vi "ConfigureChannelTrigger.vi"(8 "Error In":errorcluster, 10 "Channel Configuration":T1, 11 "Keithley 7001 In":refnum<visa-resource-name>) -> (0 "Error Out":errorcluster, 3 "Keithley 7001 Out":refnum<visa-resource-name>)   [LabVIEW 2012]
uses:
  TriggerChannelConfiguration.ctl
  driver/Public/Controls/TriggerSource.ctl
  driver/Keithley-7001.lvlib
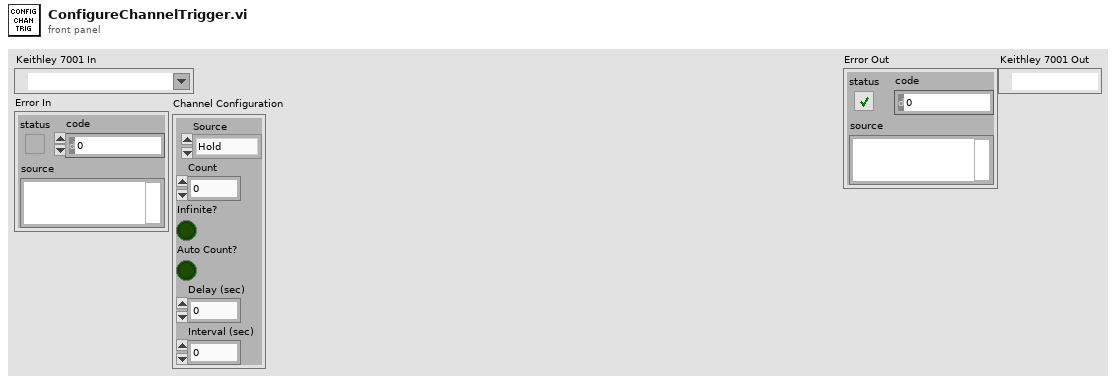
[diagram p1: front panel]
types:
  T1 = typedef "TriggerChannelConfiguration.ctl" = cluster{"Source":T2, "Count":u32, "Infinite?":bool, "Auto Count?":bool, "Delay (sec)":dbl, "Interval (sec)":dbl}
  T2 = typedef "Keithley-7001.lvlib/TriggerSource.ctl" = enum16{"Hold", "Immediate", "Manual", "Bus", "TLink", "External", "Timer"}
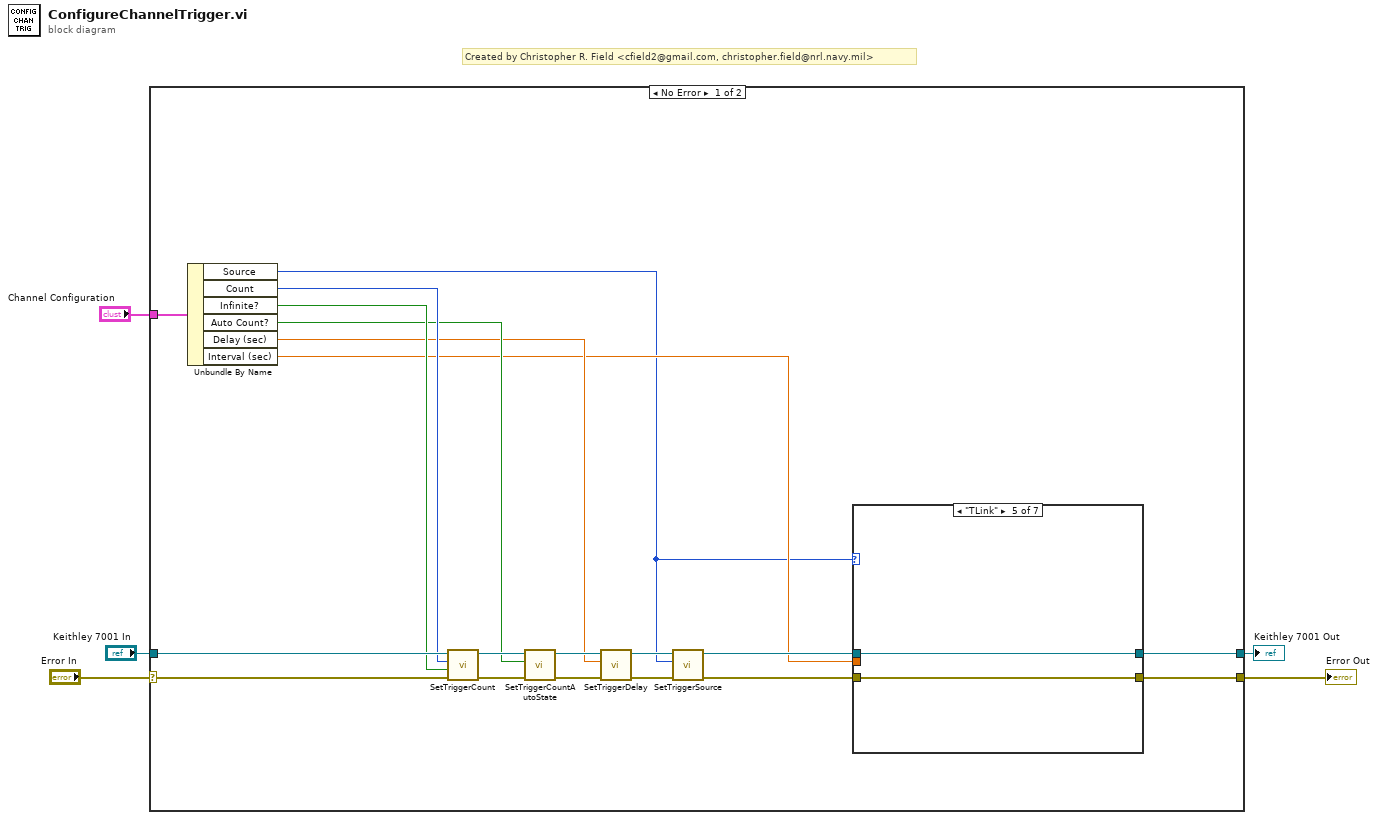
[diagram p0: block diagram]
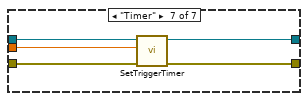
[diagram p7: hidden frame]
diagram:
  # "Created by Christopher R. Field <cfield2@gmail.com, christopher.field@nrl.navy.mil>"
  n1 = case shown="No Error" "Error In" {
    selector: "Error In" -> [w15 w42]
    tunnel: "Keithley 7001 In" -> [w16 w43]
    tunnel: [w6 w42] -> w3
    tunnel: [w7 w43] -> w2
    tunnel: "Channel Configuration" -> [w14 _]
    frame No Error {
      n2 = Unbundle By Name(w14) -> ("Source"=w8:T2, "Count"=w13:u32, "Infinite?"=w12:bool, "Auto Count?"=w11:bool, "Delay (sec)"=w10:dbl, "Interval (sec)"=w9:dbl)
      n3 = call "SetTriggerCount.vi"("Error In"=w15, "Infinite?"=w12, "Count (1-9999)"=w13, "Keithley 7001 In"=w16) -> ("Error Out"=w24:errorcluster, "Keithley 7001 Out"=w23:refnum<visa-resource-name>)  [unwired: 6 in]
      n4 = call "SetTriggerCountAutoState.vi"("Error In"=w24, "Auto?"=w11, "Keithley 7001 In"=w23) -> ("Error Out"=w21:errorcluster, "Keithley 7001 Out"=w22:refnum<visa-resource-name>)  [unwired: 7 in]
      n5 = call "SetTriggerDelay.vi"("Error In"=w21, "Delay (sec)"=w10, "Keithley 7001 In"=w22) -> ("Error Out"=w20:errorcluster, "Keithley 7001 Out"=w19:refnum<visa-resource-name>)  [unwired: 7 in]
      n6 = call "SetTriggerSource.vi"("Error In"=w20, "Source"=w8, "Keithley 7001 In"=w19) -> ("Error Out"=w18:errorcluster, "Keithley 7001 Out"=w17:refnum<visa-resource-name>)  [unwired: 7 in]
      n7 = case shown="\"TLink\"" w8 {
        tunnel: w18 -> [w25 w27 w29 w31 w33 w35 w39]
        tunnel: w17 -> [w26 w28 w30 w32 w34 w36 w41]
        tunnel: w9 -> [_ _ _ _ _ _ w40]
        tunnel: [w26 w28 w30 w32 w34 w36 w37] -> w7
        tunnel: [w25 w27 w29 w31 w33 w35 w38] -> w6
        frame "Hold", Default {
        }
        frame "Immediate" {
        }
        frame "Manual" {
        }
        frame "Bus" {
        }
        frame "TLink" {
        }
        frame "External" {
        }
        frame "Timer" {
          n8 = call "SetTriggerTimer.vi"("Error In"=w39, "Interval (sec)"=w40, "Keithley 7001 In"=w41) -> ("Error Out"=w38:errorcluster, "Keithley 7001 Out"=w37:refnum<visa-resource-name>)  [unwired: 7 in]
        }
      }
    }
    frame Error {
    }
  }
  "Error Out" <- w3
  "Keithley 7001 Out" <- w2
